vi "send_manipulatorJump-v02.vi"(0 "daq_ao 2":tag="Dev1/ao1", 1 "Duration (s)":dbl, 2 "controls array in":refnum<vi>[](array[refnum]), 3 "Sample Freq (Hz)":dbl min=0.0 max=40000.0, 4 "Phase":dbl, 5 "Duty Cycle":dbl, 6 "daq_ai":tag="Dev1/ai0:1", 8 "Use Current Position for Start Pos?":bool, 9 "Number of Replicates":i16=1 min=1 max=10, 10 "Start Position":T2(ring), 11 "common cluster":T3, 12 "Jump Position":T2(ring), 13 "error in":errorcluster) -> (14 "output cluster":T1={"daq_ao 2"="", "Duration (s)"=0.0, "Sample Freq (Hz)"=0.0, "Phase"=0.0, "Duty Cycle"=0.0, "Jump Filter Freq (Hz)"=0.0, "Number of Replicates"=1} {"Number of Replicates" min=1 max=10}, 16 "control array out":refnum<vi>[](array[refnum]), 17 "protcol waveform":waveform(dbl)(graph), 18 "error out":errorcluster, 19 "protcol response":waveform(dbl)[](graph) caption="jumptestMonitor")   [LabVIEW 2019]
uses:
  multipatch/controls/multipatch_common_controls_v4.ctl
  machine_vision/controls/transform_cluster_actuator.ctl
  machine_vision/coordinate model vis/transform_properties_actuators.ctl
  pipette cleaning/pressure box/cleaning_soft/controls/actuator_cluster.ctl
  pipette cleaning/pressure box/cleaning_soft/controls/actuator_type.ctl
  pipette cleaning/pressure box/cleaning_soft/controls/pressure_box_control.ctl
  pipette cleaning/pressure box/cleaning_soft/controls/pressure_box_type.ctl
  controls/NH_method.ctl
  <vilib>/measure/NI_MABase.lvlib
panel:
  in  "Jump Filter Freq (Hz)":dbl=20.0 min=0.0 max=40000.0
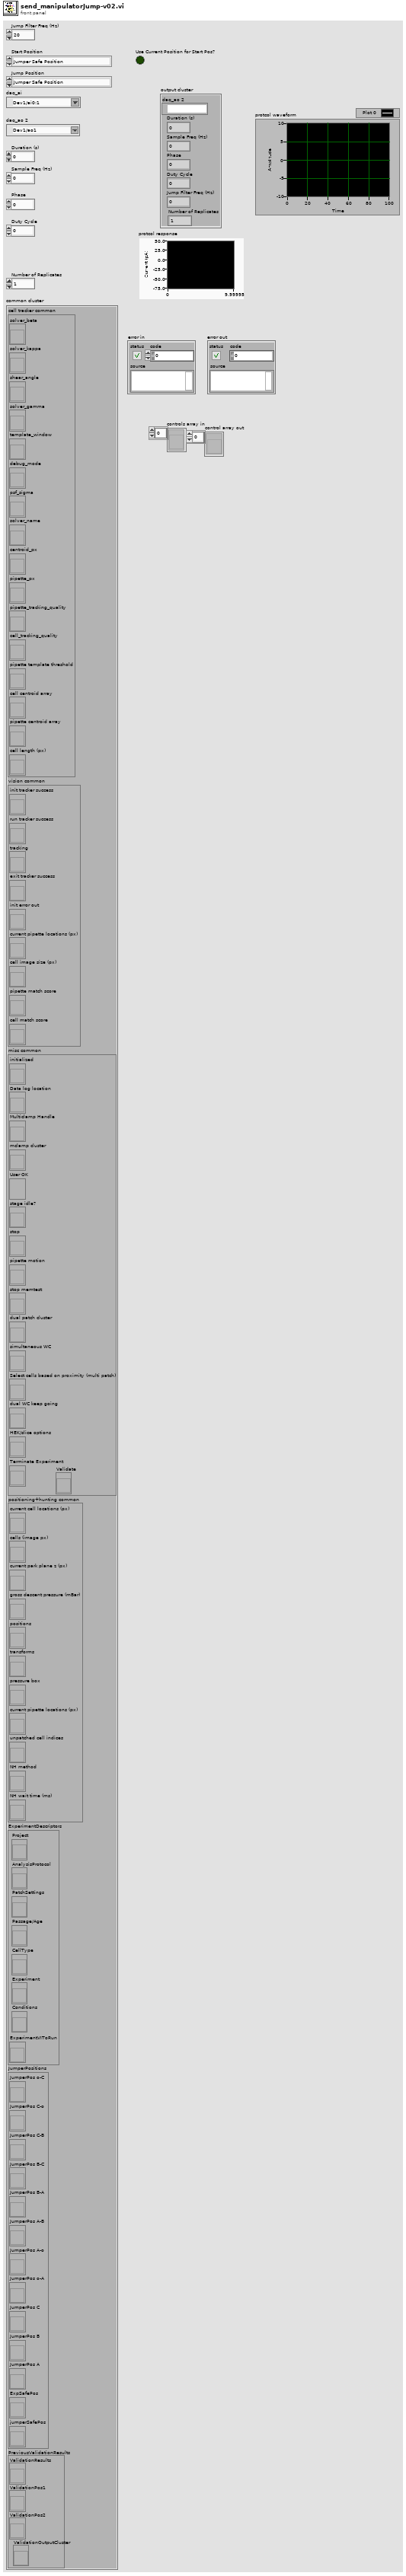
[diagram p1: front panel]
types:
  T1 = cluster{"daq_ao 2":tag, "Duration (s)":dbl, "Sample Freq (Hz)":dbl, "Phase":dbl, "Duty Cycle":dbl, "Jump Filter Freq (Hz)":dbl, "Number of Replicates":i16}
  T2 = enum16{"Jumper Safe Position", "Experiment Safe Position", "Jumper Position A", "Jumper Position B", "Jumper Position C", "Jumper Position o-A", "Jumper Position A-o", "Jumper Position A-B", "Jumper Position B-A", "Jumper Position B-C", "Jumper Position C-B", "Jumper Position C-o", "Jumper Position o-C"}
  T3 = typedef "multipatch_common_controls_v4.ctl" = cluster{"cell tracker common":cluster{"solver_beta":refnum<vi>, "solver_kappa":refnum<vi>, "shear_angle":refnum<vi>, "solver_gamma":refnum<vi>, "template_window":refnum<vi>, "debug_mode":refnum<vi>, "psf_sigma":refnum<vi>, "solver_name":refnum<vi>, "centroid_px":refnum<vi>, "pipette_px":refnum<vi>, "pipette_tracking_quality":refnum<vi>, "cell_tracking_quality":refnum<vi>, "pipette template threshold":refnum<vi>, "cell centroid array":refnum<vi>, "pipette centroid array":refnum<vi>, "cell length (px)":refnum<vi>}, "vision common":cluster{"init tracker success":refnum<vi>, "run tracker success":refnum<vi>, "tracking":refnum<vi>, "exit tracker success":refnum<vi>, "init error out":refnum<vi>, "current pipette locations (px)":refnum<vi>, "cell image size (px)":refnum<vi>, "pipette match score":refnum<vi>, "cell match score":refnum<vi>}, "misc common":cluster{"initialized":refnum<vi>, "Data log location":refnum<vi>, "Multiclamp Handle":refnum<vi>, "mclamp cluster":refnum<vi>, "User OK":refnum<vi>, "stage idle?":refnum<vi>, "stop":refnum<vi>, "pipette motion":refnum<vi>, "stop memtest":refnum<vi>, "dual patch cluster":refnum<vi>, "simultaneous WC":refnum<vi>, "Select cells based on proximity (multi patch)":refnum<vi>, "dual WC keep going":refnum<vi>, "HEK/slice options":refnum<vi>, "Terminate Experiment":refnum<vi>, "Validate":refnum<vi>}, "positioning+hunting common":cluster{"current cell locations (px)":refnum<vi>, "cells (image px)":refnum<vi>, "current park plane z (px)":refnum<vi>, "gross descent pressure (mBar)":refnum<vi>, "positions":refnum<vi>, "transforms":refnum<vi>, "pressure box":refnum<vi>, "current pipette locations (px)":refnum<vi>, "unpatched cell indices":refnum<vi>, "NH method":refnum<vi>, "NH wait time (ms)":refnum<vi>}, "ExperimentDescriptors":cluster{"Project":refnum<vi>, "AnalysisProtocol":refnum<vi>, "PatchSettings":refnum<vi>, "Passage/Age":refnum<vi>, "CellType":refnum<vi>, "Experiment":refnum<vi>, "Conditions":refnum<vi>, "ExperimentVIToRun":refnum<vi>}, "JumperPositions":cluster{"JumperPos o-C":refnum<vi>, "JumperPos C-o":refnum<vi>, "JumperPos C-B":refnum<vi>, "JumperPos B-C":refnum<vi>, "JumperPos B-A":refnum<vi>, "JumperPos A-B":refnum<vi>, "JumperPos A-o":refnum<vi>, "JumperPos o-A":refnum<vi>, "JumperPos C":refnum<vi>, "JumperPos B":refnum<vi>, "JumperPos A":refnum<vi>, "ExpSafePos":refnum<vi>, "jumperSafePos":refnum<vi>}, "PreviousValidationResults":cluster{"ValidationResults":refnum<vi>, "ValidationPos1":refnum<vi>, "ValidationPos2":refnum<vi>, "ValidationOutputCluster":refnum<vi>}}
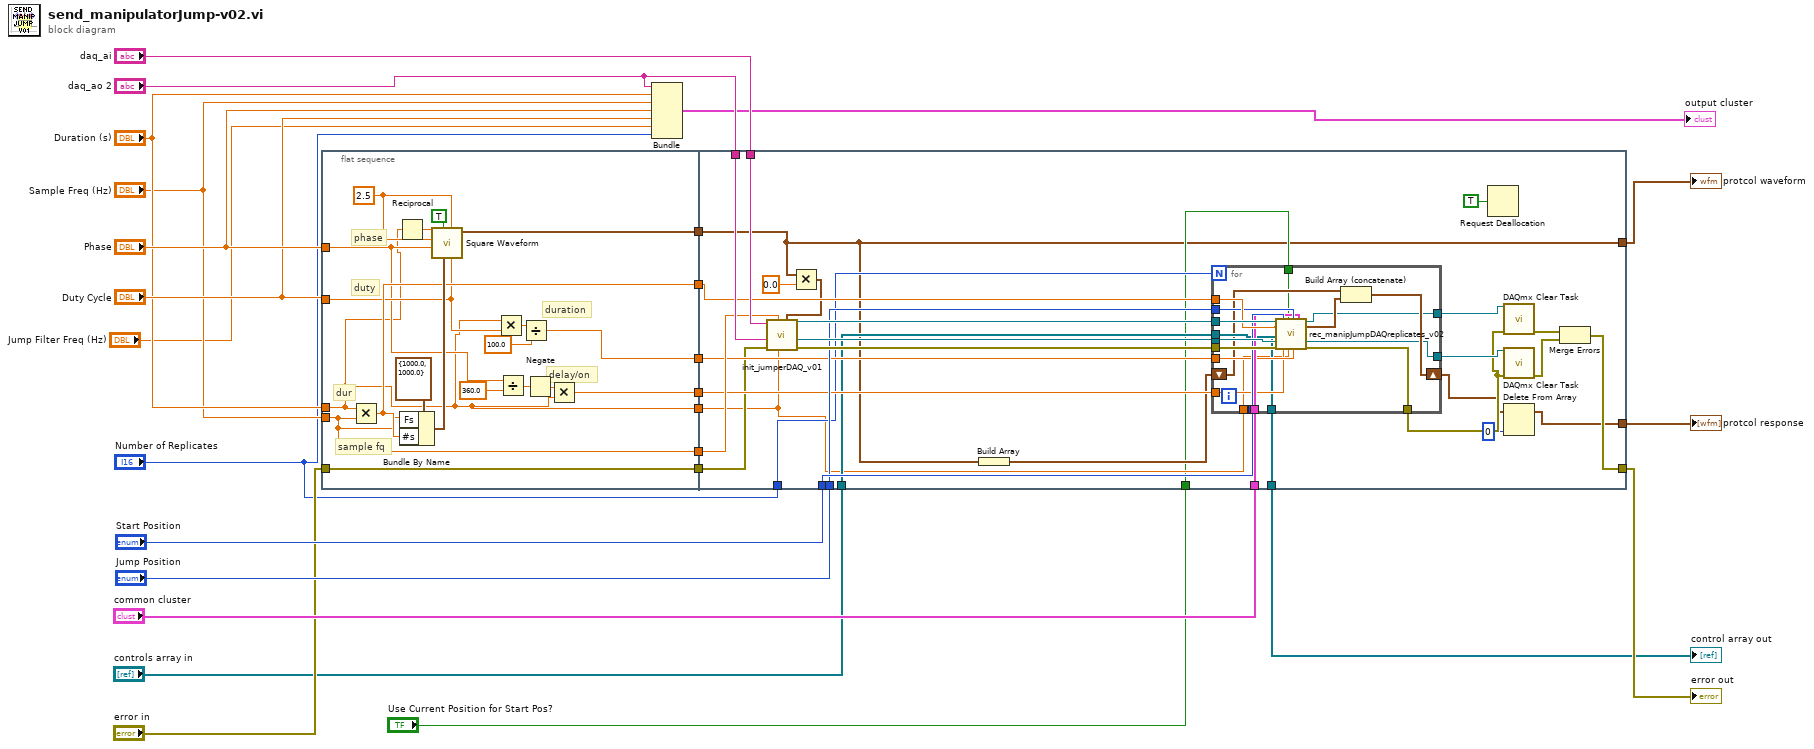
[diagram p0: block diagram]
diagram:
  n1 = flat-sequence {
    tunnel: "Phase" -> [w35]
    tunnel: "Duty Cycle" -> [w38]
    tunnel: "Duration (s)" -> [w27]
    tunnel: "Sample Freq (Hz)" -> [w40]
    tunnel: [w41] -> w18
    tunnel: [w40] -> w16
    tunnel: [w39] -> w17
    tunnel: [w31] -> w12
    tunnel: [w30] -> w11
    tunnel: "error in" -> [w28]
    tunnel: [w28] -> w9
    tunnel: [w27] -> w2
    tunnel: [w46] -> w23
    tunnel: w18 -> [w71]
    tunnel: w17 -> [w46]
    tunnel: "daq_ai" -> [w74]
    tunnel: "daq_ao 2" -> [w73]
    tunnel: w16 -> [w72]
    tunnel: [w51] -> w20
    tunnel: "Number of Replicates" -> [w61]
    tunnel: "Start Position" -> [w68]
    tunnel: "Jump Position" -> [w67]
    tunnel: "common cluster" -> [w66]
    tunnel: w12 -> [w65]
    tunnel: w11 -> [w64]
    tunnel: [w55] -> w8
    tunnel: w9 -> [w60]
    tunnel: "controls array in" -> [w63]
    tunnel: [w62] -> w6
    tunnel: w2 -> [w49]
    tunnel: "Use Current Position for Start Pos?" -> [w48]
    frame #0 {
      w45 = 2.5 ("Amplitude")
      # "sample fq"
      # "dur"
      # "duty"
      # "phase"
      # "delay/on"
      # "duration"
      n2 = Multiply(x=w27, y=w40) -> (x*y=w41:dbl)
      n3 = Reciprocal(x=w27) -> (1/x=w29:dbl)
      n4 = Bundle By Name(cluster=cluster{"Fs":dbl, "#s":dbl} {"Fs"=1000.0, "#s"=1000.0} ("sampling info"), "Fs"=w40, "#s"=w41) -> (w42:cluster{"Fs":dbl, "#s":dbl})
      n5 = call <vilib>:"Square Waveform.vi"("duty cycle (%)"=w38, "offset"=w45, "sampling info"=w42, "reset signal"=TRUE, "phase"=w35, "amplitude"=w45, "frequency"=w29) -> ("signal out"=w39:waveform(dbl))  [unwired: 3 in, 1 out]
      n6 = Multiply(x=w27, y=w38) -> (x*y=w37:dbl)
      n7 = Divide(x=w35, y=360.0) -> (x/y=w33:dbl)
      n8 = Divide(x=w37, y=100.0) -> (x/y=w31:dbl)
      n9 = Negate(x=w33) -> (-x=w32:dbl)
      n10 = Multiply(x=w32, y=w27) -> (x*y=w30:dbl)
    }
    frame #1 {
      n11 = Multiply(x=w46, y=0.0) -> (x*y=w69:waveform(dbl))
      n12 = call "init_jumperDAQ_v01.vi"("protocol waveform"=w69, "Duration (s)"=w49, "Sample Freq (Hz)"=w72, "AO error in"=w60, "AO physical channels"=w73, "AI Physical Channel"=w74) -> ("AO error out"=w77:errorcluster, "AO task out"=w76:refnum<k21>, "AI task out"=w75:refnum<k21>)  [unwired: 1 in, 2 out]
      n13 = Build Array(w46) -> (w53:waveform(dbl)[])
      n14 = for {
        N: w61 -> [_]
        tunnel: w77 -> [w96]
        tunnel: w76 -> [w95]
        tunnel: w75 -> [w94]
        tunnel: w71 -> [w92]
        tunnel: w68 -> [w91]
        tunnel: w67 -> [w90]
        tunnel: w66 -> [w89]
        tunnel: w65 -> [w88]
        tunnel: w64 -> [w87]
        tunnel: w63 -> [w86]
        tunnel: [w85] -> w62
        shift-right: [w84] -> w52
        shift-left: w53 -> [w82]
        tunnel: [w93] -> w57
        tunnel: [w81] -> w59
        tunnel: [w80] -> w58
        tunnel: w49 -> [w79]
        tunnel: w48 -> [w78]
        n15 = call "rec_manipJumpDAQreplicates_v02.vi"("AI task in"=w94, "number of samples"=w92, "controls array in"=w86, "AO task in"=w95, "error in"=w96, "Start Position"=w91, "Jump On Time (s)"=w87, "Use Current Position for Start Pos?"=w78, "Duration (s)"=w79, "Jump Position"=w90, "Jump Duration (s)"=w88, "common cluster"=w89) -> ("AI task out"=w80:refnum<k21>, "data out (pA or mV)"=w83:waveform(dbl), "control array out"=w85:refnum<vi>[], "AO task out"=w81:refnum<k21>, "error out"=w93:errorcluster)  [unwired: 3 in]
        n16 = Build Array (concatenate)(w82, w83) -> (w84:waveform(dbl)[])
      }
      n17 = Request Deallocation(TRUE ("flag")) -> ()
      n18 = call <vilib>:"DAQmx Clear Task.vi"("task in"=w58, "error in"=w57) -> ("error out"=w54:errorcluster)  [unwired: 13 in]
      n19 = call <vilib>:"DAQmx Clear Task.vi"("task in"=w59, "error in"=w57) -> ("error out"=w56:errorcluster)  [unwired: 13 in]
      n20 = Delete From Array(array=w52, index=0) -> (array with subset deleted=w51:waveform(dbl)[])  [unwired: 1 in, 1 out]
      n21 = Merge Errors(w54, w56) -> (w55:errorcluster)
    }
  }
  n22 = Bundle("daq_ao 2"="daq_ao 2", "Duration (s)"="Duration (s)", "Sample Freq (Hz)"="Sample Freq (Hz)", "Phase"="Phase", "Duty Cycle"="Duty Cycle", "Jump Filter Freq (Hz)"="Jump Filter Freq (Hz)", "Number of Replicates"="Number of Replicates") -> (→"output cluster":T1)  [unwired: 1 in]
  "protcol response" <- w20
  "protcol waveform" <- w23
  "error out" <- w8
  "control array out" <- w6
